vi "Create Arm.vi"(6 "Length":sgl, 9 "Name":string, 10 "Color":cluster{"R":sgl, "G":sgl, "B":sgl, "A":sgl}, 11 "Radius":sgl) -> (1 "Half Length":sgl, 2 "Transformation.GetTranslation":T1, 3 "SceneObject out":refnum<vi>)   [LabVIEW 2021]
uses:
  <vilib>/Utility/miscctls.llb/LV3DPointTypeDef.ctl
  <vilib>/picture/3D Picture Control/Object/Create Object (drawable).vi
  <vilib>/picture/3D Picture Control/NI_3D Picture Control.lvlib
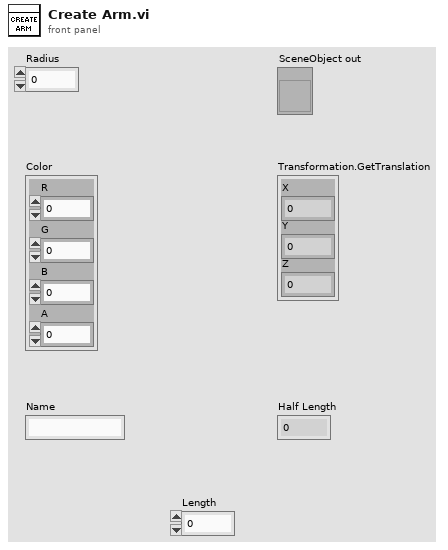
[diagram p1: front panel]
types:
  T1 = typedef "LV3DPointTypeDef.ctl" = cluster{"X":sgl, "Y":sgl, "Z":sgl}
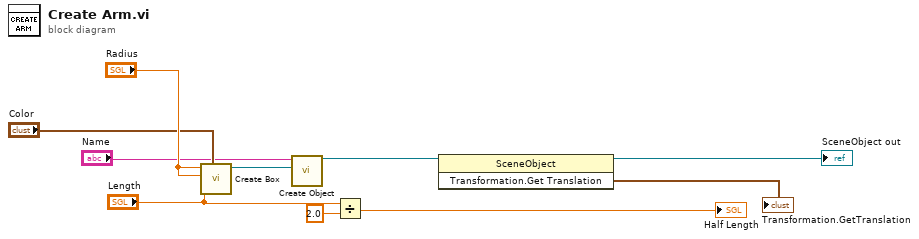
[diagram p0: block diagram]
diagram:
  n1 = call <vilib>:"Create Box.vi"("Color"="Color", "Length Z"="Length", "Length Y"="Radius", "Length X"="Radius") -> ("New Box Refnum"=w2:refnum<vi>)  [unwired: 6 in, 1 out]
  n2 = call-poly <vilib>:"Create Object.vi"("Geometry"=w2, "Name"="Name") -> ("Scene:New Object"=w3:refnum<vi>)  [unwired: 8 in, 1 out]
  n3 = Divide(x="Length", y=sgl 2.0) -> (x/y=→"Half Length":sgl)
  n4 = invoke class="SceneObject" method="Transformation.Get Translation"(reference=w3) -> (reference out=→"SceneObject out":refnum<vi>, "Transformation.GetTranslation"=→"Transformation.GetTranslation":T1)  [unwired: 2 in, 1 out]
